vi "Set File Attributes.vi"(8 "error in (no error)":errorcluster, 9 "Action (\"-R +A -H\")":string="-R +A -H", 10 "File Name (\"D:\\user\\data\")":string="D:\\user\\data", 11 "VISA resource name":refnum<visa-resource-name>) -> (0 "error out":errorcluster, 3 "VISA resource name out":refnum<visa-resource-name>)   [LabVIEW 2020, in "Rohde&Schwarz CMXP Base.lvlib"]
doc: "Sets file properties for files and directories.\n\nAttribute:\nRSCMXPBASE_ATTR_SET_FILE_ATTRIBUTE\n\nRemote-control command:\nMMEMory:ATTRibute"
uses:
  <instrlib>/Rohde&Schwarz CMXP Base/Rohde&Schwarz CMXP Base.lvlib
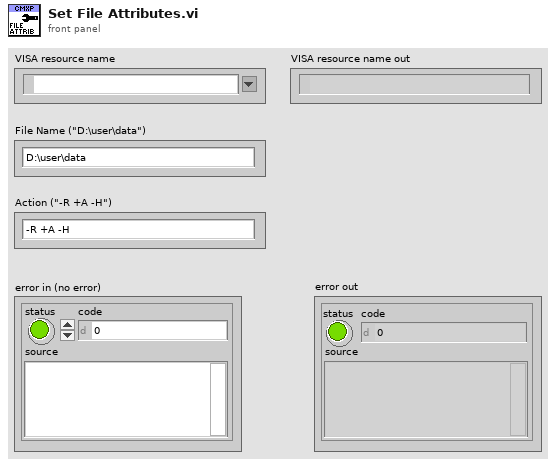
[diagram p1: front panel]
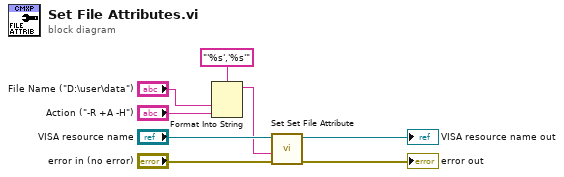
[diagram p0: block diagram]
diagram:
  n1 = Format Into String(format string="'%s','%s'", "File Name (\"D:\\user\\data\")", "Action (\"-R +A -H\")") -> (resulting string=w1:string)  [unwired: 2 in, 1 out]
  n2 = call "Set Set File Attribute"("error in (no error)"="error in (no error)", "Set File Attribute ()"=w1, "instrument handle"="VISA resource name") -> ("error out"=→"error out":errorcluster, "instrument handle out"=→"VISA resource name out":refnum<visa-resource-name>)  [unwired: 7 in]
